vi "XY graphs.vi"() -> ()   [LabVIEW 2024]
uses:
  <vilib>/numeric/Random Number (Range) DBL.vi
panel:
  out "XY Graph":cluster{i32[], dbl[]}(graph)
  out "Waveform Graph":dbl[](graph)
  out "Array":dbl[](array[numeric])
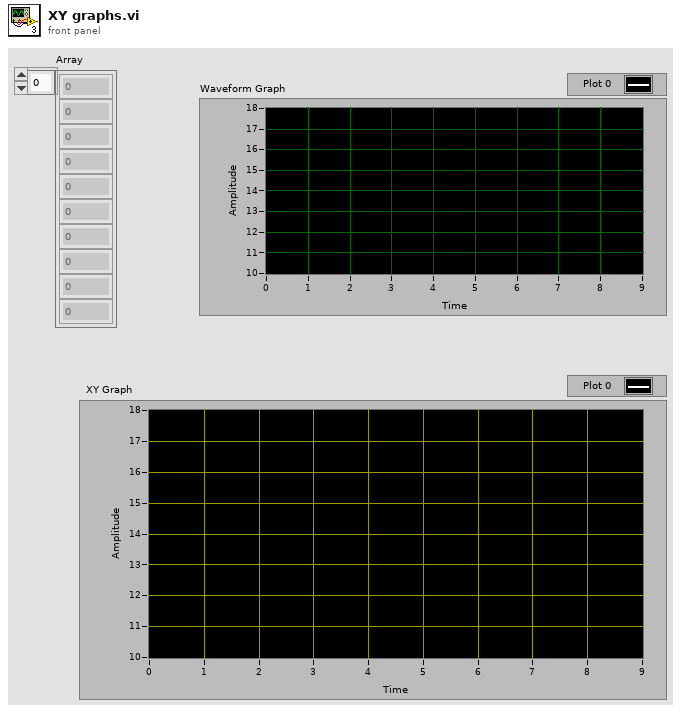
[diagram p1: front panel]
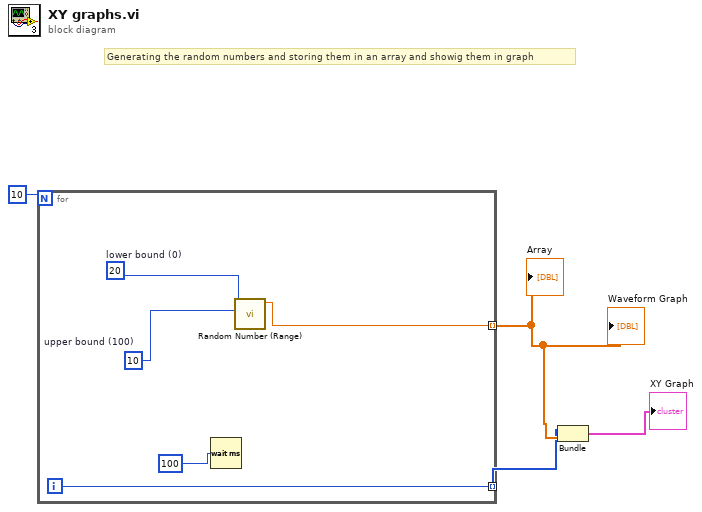
[diagram p0: block diagram]
diagram:
  # "Generating the random numbers and storing them in an array and showig them in graph"
  n1 = for {
    N: 10 -> [_]
    tunnel: [w6] -> w2 mode=indexing
    tunnel: [w5] -> w1 mode=indexing
    i -> [w5]
    w7 = u64 10  # upper bound (100)
    w9 = u64 20  # lower bound (0)
    n2 = Wait (ms)(milliseconds to wait=u32 100 ("millisecond timer value")) -> ()  [unwired: 1 out]
    n3 = call-poly <vilib>:"Random Number (Range).vi"("lower bound (0)"=w7, "upper bound (100)"=w9) -> ("number"=w6:dbl)  [unwired: 9 in]
  }
  "Array" <- w2
  "Waveform Graph" <- w2
  n4 = Bundle(w1, w2) -> (→"XY Graph":cluster{i32[], dbl[]})  [unwired: 1 in]
